vi "TestVI.vi"() -> ()   [LabVIEW 2020]
uses:
  DMM/DMM.lvclass/DMM.ctl
  DMM/Read Range.vi
  DMM/DMM.lvclass
panel:
  out "Range 2":dbl
  in  "Scale":enum16{"1u", "1m", "1", "10", "100", "1k", "1M"}(ring)
  in  "Range":dbl
  in  "Measurement Type":enum16{"DCV", "ACV", "DCI", "ACI"}(ring)
  in  "DMM Alias":string
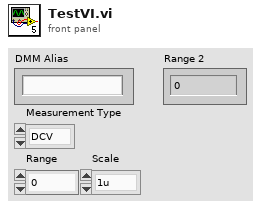
[diagram p1: front panel]
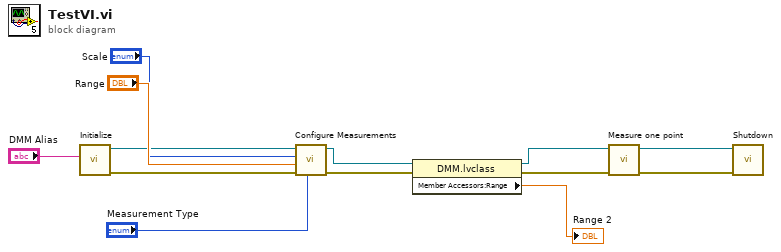
[diagram p0: block diagram]
diagram:
  n1 = call "Initialize.vi"("DMM Alias"="DMM Alias") -> ("error out"=w13:errorcluster, "DMM out"=w5:refnum<class "DMM.lvclass">)  [unwired: 9 in]
  n2 = call "Configure Measurements.vi"("Measurement Type"="Measurement Type", "error in (no error)"=w13, "Range"="Range", "Scale"="Scale", "DMM in"=w5) -> ("error out"=w12:errorcluster, "DMM out"=w3:refnum<class "DMM.lvclass">)  [unwired: 5 in]
  n3 = property class="DMM.lvclass"(reference=w3, error in=w12) -> (reference out=w2:refnum<class "DMM.lvclass">, error out=w4:errorcluster, "Member Accessors:Range"=→"Range 2":dbl)
  n4 = call "Measure one point.vi"("error in (no error)"=w4, "DMM in"=w2) -> ("error out"=w11:errorcluster, "DMM out"=w10:refnum<class "DMM.lvclass">)  [unwired: 8 in]
  n5 = call "Shutdown.vi"("error in (no error)"=w11, "DMM in"=w10) -> ()  [unwired: 8 in, 2 out]
